vi "SFTP File Type - invalid file type - returns Unknown.vi"() -> ()   [LabVIEW 2017, in "unit_tests.lvlib"]
uses:
  unit_tests.lvlib
  libssh2/SFTP File Type.ctl
  libssh2/libssh2.lvlib
  <vilib>/PNR/Transparent Assertions/Transparent Assertions/Transparent Assertions.lvlib
panel:
  out "error out":errorcluster
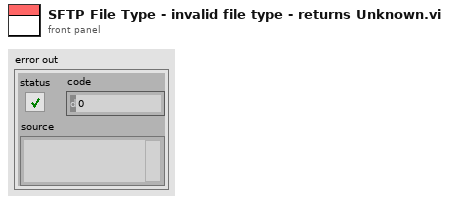
[diagram p1: front panel]
types:
  T1 = typedef "libssh2.lvlib/SFTP File Type.ctl" = enum16{"Unknown", "Named Pipe (FIFO)", "Character Special File", "Directory", "Block Special File", "Regular File", "Symbolic Link", "Socket"}
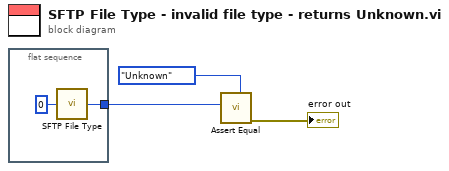
[diagram p0: block diagram]
diagram:
  n1 = flat-sequence {
    tunnel: [w5] -> w1
    frame #0 {
      n2 = call "SFTP File Type.vi"("permissions"=u32 0) -> ("type"=w5:T1)
    }
  }
  n3 = call <vilib>:"Assert Equal.vi"("Expected"=SFTP_File_Type."Unknown" ("type"), "Actual"=w1) -> ("error out"=→"error out":errorcluster)  [unwired: 9 in]
